vi "Set Control Panel Data.vi"(8 "error in (no error)":errorcluster, 10 "Data":variant, 11 "Device in":refnum<class "Device.lvclass">) -> (0 "error out":errorcluster, 3 "Device out":refnum<class "Device.lvclass">)   [LabVIEW 2015, in "Device.lvclass"]
uses:
  Device.lvclass
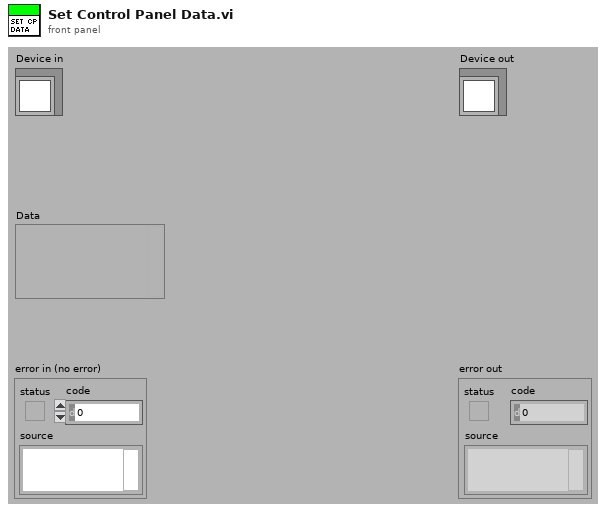
[diagram p1: front panel]
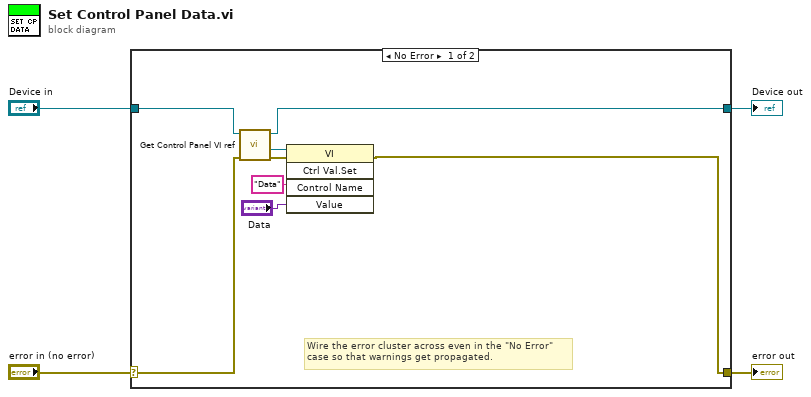
[diagram p0: block diagram]
diagram:
  n1 = case shown="No Error" "error in (no error)" {
    selector: "error in (no error)" -> [w7 w14]
    tunnel: [w6 w14] -> w3
    tunnel: [w8 w13] -> w1
    tunnel: "Device in" -> [w9 w13]
    frame No Error {
      # "Wire the error cluster across even in the \"No Error\"\ncase so that warnings get propagated."
      n2 = call "Get Control Panel VI ref.vi"("error in (no error)"=w7, "Device in"=w9) -> ("error out"=w11:errorcluster, "vi ref out"=w10:refnum<vi>, "Device out"=w8:refnum<class "Device.lvclass">)  [unwired: 7 in]
      n3 = invoke class="VI" method="Ctrl Val.Set"(reference=w10, error in=w11, "Control Name"="Data", "Value"="Data") -> (error out=w6:errorcluster)  [unwired: 1 in, 4 out]
    }
    frame Error {
    }
  }
  "error out" <- w3
  "Device out" <- w1
